vi "parseCustomFlag2_REAL.vi"(8 "error in (no error)":errorcluster, 10 "Numeric":i8, 11 "OrionBMS in":refnum<class "OrionBMSClass.lvclass">) -> (0 "error out":errorcluster, 2 "output cluster":T1, 3 "OrionBMS out":refnum<class "OrionBMSClass.lvclass">)   [LabVIEW 2018, in "OrionBMSClass.lvclass"]
uses:
  OrionBMSClass.lvclass
  Type_Def/TypeDef_BMSStatuss.ctl
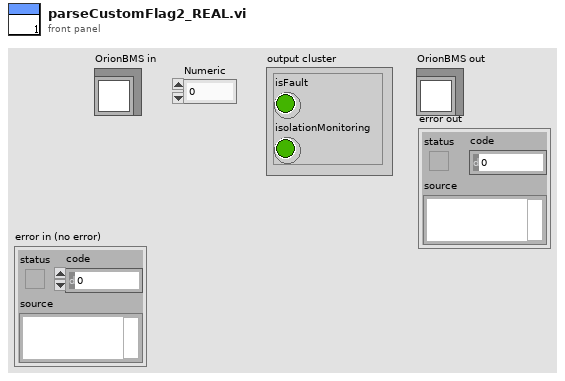
[diagram p1: front panel]
types:
  T1 = typedef "TypeDef_BMSStatuss.ctl" = cluster{"isFault":bool, "isolationMonitoring":bool}
  T2 = typedef "TypeDef_BMSDatas.ctl" = cluster{"Pack 1 Max Cell\n Voltage (V)":dbl, "Pack 1 Max Cell\n ID ":dbl, "Pack 1 Min Cell \nVoltage (V)":dbl, "Pack 1 Min Cell \nID ":dbl, "Pack 1 State of Charge  (%)":dbl, "Pack 1 Average Voltage1 (V)":dbl, "Pack 1Voltage Delta (V)":dbl, "Pack 1 Current (A)":dbl, "Pack 1 Voltage (V)":dbl, "Pack 1 Max Resistance (Ohm)":dbl, "Pack 1Min Resistance (Ohm)":dbl, "Pack 1Average Resistance (Ohm)":dbl, "Pack 1Delta Resistance (Ohm)":dbl, "Pack 1 Highest Temperature(F)":dbl, "BmsStatus1":T1, "Pack 2 Max Cell\n Voltage (V) ":dbl, "Pack 2 Max Cell\n ID  ":dbl, "Pack 2 Min Cell \nVoltage (V) ":dbl, "Pack 2 Min Cell \nID  ":dbl, "Pack 2 Average Voltage1 (V)":dbl, "Pack 2 Voltage Delta (V) ":dbl, "Pack 2 Current (A)":dbl, "Pack 2 Voltage (V) ":dbl, "Pack 2 State of Charge  (%) ":dbl, "Pack 2 Max Resistance (Ohm) ":dbl, "Pack 2 Min Resistance (Ohm)":dbl, "Pack 2 Average Resistance (Ohm)":dbl, "Pack 2 Delta Resistance (Ohm) ":dbl, "Pack 2 Highest Temperature(F) ":dbl, "BmsStatus 2":T1}
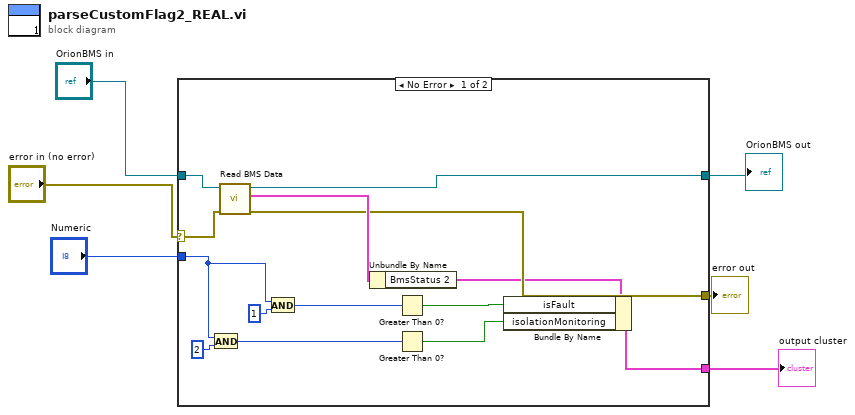
[diagram p0: block diagram]
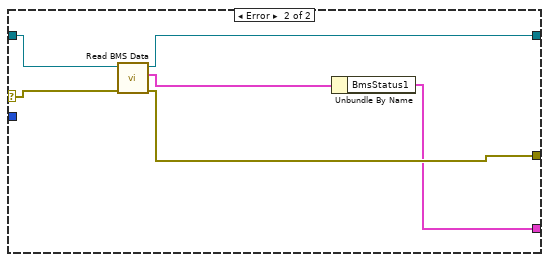
[diagram p2: hidden frame]
diagram:
  n1 = case shown="No Error" "error in (no error)" {
    selector: "error in (no error)" -> [w14 w25]
    tunnel: "OrionBMS in" -> [w20 w26]
    tunnel: [w19 w24] -> w2
    tunnel: [w13 w23] -> w4
    tunnel: "Numeric" -> [w17 _]
    tunnel: [w7 w21] -> w6
    frame No Error {
      n2 = And(x=w17, y=2) -> (x .and. y?=w10:i32)
      n3 = call-dynamic "Read BMS Data.vi"("error in (no error)"=w14, "OrionBMS in"=w20) -> ("error out"=w13:errorcluster, "BMS Data"=w15:T2, "OrionBMS out"=w19:refnum<class "OrionBMSClass.lvclass">)  [unwired: 7 in]
      n4 = And(x=w17, y=1) -> (x .and. y?=w11:i32)
      n5 = Unbundle By Name(w15) -> ("BmsStatus 2"=w12:T1)
      n6 = Greater Than 0?(x=w11) -> (x > 0?=w9:bool)
      n7 = Greater Than 0?(x=w10) -> (x > 0?=w8:bool)
      n8 = Bundle By Name(cluster=w12, "isFault"=w9, "isolationMonitoring"=w8) -> (w7:T1)
    }
    frame Error {
      n9 = call-dynamic "Read BMS Data.vi"("error in (no error)"=w25, "OrionBMS in"=w26) -> ("error out"=w23:errorcluster, "BMS Data"=w22:T2, "OrionBMS out"=w24:refnum<class "OrionBMSClass.lvclass">)  [unwired: 7 in]
      n10 = Unbundle By Name(w22) -> ("BmsStatus1"=w21:T1)
    }
  }
  "OrionBMS out" <- w2
  "error out" <- w4
  "output cluster" <- w6
